vi "Main PC.vi"() -> ()   [LabVIEW 2015]
panel:
  out "Debug mode":bool
  out "Ipad mode":bool
  out "Keyboard mode":bool
  in  "?":bool
  out "?":u32(colorbox)
  out "?":u32(colorbox)
  out "?":u32(colorbox)
  out "?":u32(colorbox)
  out "Speed  1":bool
  out "Speed 3":bool
  out "Speed 2":bool
  out "MD49 driver response":string
  in  "Send command":string
  in  "Debug mode":bool
  in  "Keyboard Mode":bool
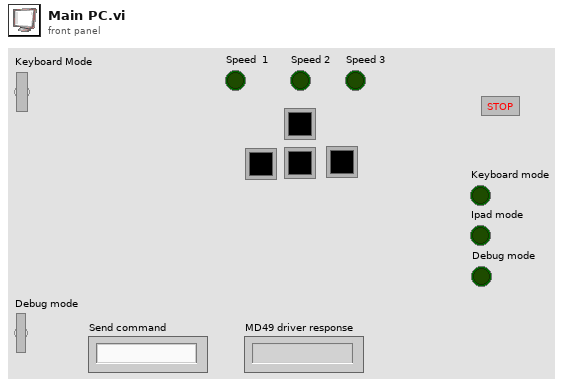
[diagram p1: front panel]
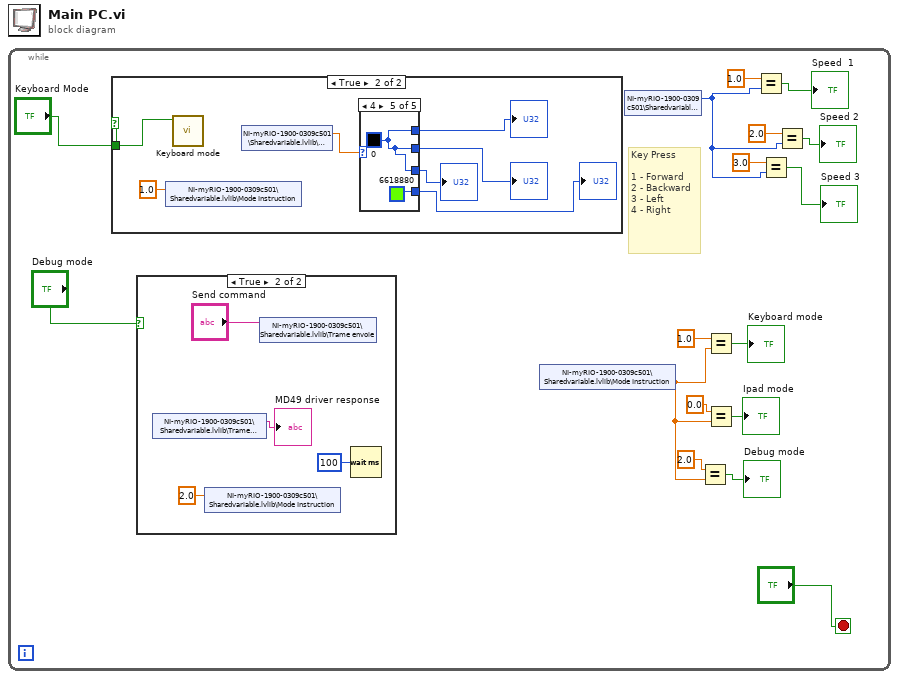
[diagram p0: block diagram]
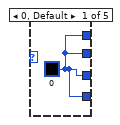
[diagram p3: hidden frame]
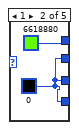
[diagram p4: hidden frame]
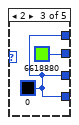
[diagram p5: hidden frame]
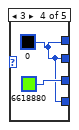
[diagram p6: hidden frame]
diagram:
  n1 = while {
    stop <- "?" stop-if-true
    # "Key Press\n\n1 - Forward\n2 - Backward\n3 - Left\n4 - Right"
    n2 = case shown="True" "Keyboard Mode" {
      tunnel: "Keyboard Mode" -> [_ w24]
      frame False {
      }
      frame True {
        n3 = shared-variable "NI-myRIO-1900-0309c501\\Sharedvariable.lvlib\\Mode Instruction"(1.0 ("Consigne Mode")) -> ()  [unwired: 1 in, 1 out]
        n4 = call "Keyboard mode.vi"("stop"=w24) -> ()  [unwired: 11 in]
        n5 = shared-variable "NI-myRIO-1900-0309c501\\Sharedvariable.lvlib\\KeyPress"() -> (w22:dbl)  [unwired: 1 in, 1 out]
        n6 = case shown="4" w22 {
          tunnel: [w25 u32 6618880 w28 w30 w33] -> w21
          tunnel: [w25 w27 u32 6618880 w30 w33] -> w19
          tunnel: [w25 w27 w28 u32 6618880 w33] -> w18
          tunnel: [w25 w27 w28 w30 u32 6618880] -> w20
          frame 0, Default {
            w25 = u32 0
          }
          frame 1 {
            w27 = u32 0
          }
          frame 2 {
            w28 = u32 0
          }
          frame 3 {
            w30 = u32 0
          }
          frame 4 {
            w33 = u32 0
          }
        }
        "?" <- w21
        "?" <- w20
        "?" <- w19
        "?" <- w18
      }
    }
    n7 = case shown="True" "Debug mode" {
      frame False {
      }
      frame True {
        n8 = shared-variable "NI-myRIO-1900-0309c501\\Sharedvariable.lvlib\\Trame Recue"() -> (→"MD49 driver response":string)  [unwired: 1 in, 1 out]
        n9 = shared-variable "NI-myRIO-1900-0309c501\\Sharedvariable.lvlib\\Mode Instruction"(2.0 ("Consigne Mode")) -> ()  [unwired: 1 in, 1 out]
        n10 = shared-variable "NI-myRIO-1900-0309c501\\Sharedvariable.lvlib\\Trame envoie"("Send command") -> ()  [unwired: 1 in, 1 out]
        n11 = Wait (ms)(milliseconds to wait=u32 100) -> ()  [unwired: 1 out]
      }
    }
    n12 = shared-variable "NI-myRIO-1900-0309c501\\Sharedvariable.lvlib\\Mode Instruction"() -> (w6:dbl)  [unwired: 1 in, 1 out]
    n13 = shared-variable "NI-myRIO-1900-0309c501\\Sharedvariable.lvlib\\Speed"() -> (w9:u16)  [unwired: 1 in, 1 out]
    n14 = Equal?(x=2.0, y=w6) -> (x = y?=→"Debug mode":bool)
    n15 = Equal?(x=1.0, y=w6) -> (x = y?=→"Keyboard mode":bool)
    n16 = Equal?(x=0.0, y=w6) -> (x = y?=→"Ipad mode":bool)
    n17 = Equal?(x=1.0, y=w9) -> (x = y?=→"Speed  1":bool)
    n18 = Equal?(x=3.0, y=w9) -> (x = y?=→"Speed 3":bool)
    n19 = Equal?(x=2.0, y=w9) -> (x = y?=→"Speed 2":bool)
  }
